vi "testDisplay.vi"() -> ()   [LabVIEW 2017]
panel:
  out "projBounds":T1
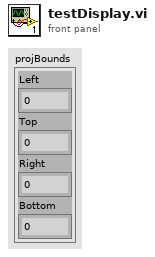
[diagram p1: front panel]
types:
  T1 = cluster{"Left":i32, "Top":i32, "Right":i32, "Bottom":i32}
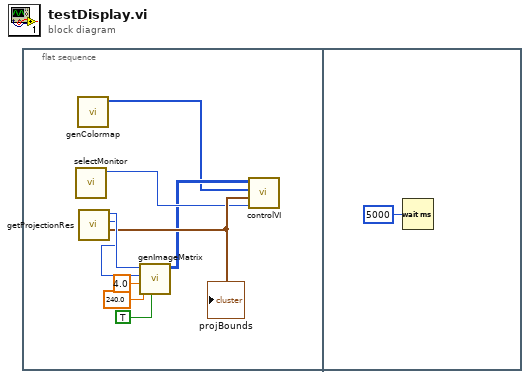
[diagram p0: block diagram]
diagram:
  n1 = flat-sequence {
    frame #0 {
      n2 = call "selectMonitor.vi"() -> ("monitor to use"=w4:i32)  [unwired: 11 in]
      n3 = call "genColormap.vi"() -> ("Colormap"=w2:u32[])  [unwired: 11 in]
      n4 = call "getProjectionRes.vi"() -> ("projBounds"=w5:T1, "YRes"=w8:i32, "XRes"=w9:i32)  [unwired: 9 in]
      "projBounds" <- w5
      n5 = call "genImageMatrix.vi"("Orientation"=TRUE, "Phase"=240.0, "Cycles"=4.0, "Y resolution"=w8, "X Resolution"=w9) -> ("Scan Image"=w3:u8[][])  [unwired: 5 in, 1 out]
      n6 = call "controlVI.vi"("monitorToUse"=w4, "Front Panel Window:Window Bounds"=w5, "colors"=w2, "8-bit pixmap"=w3) -> ()  [unwired: 7 in, 1 out]
    }
    frame #1 {
      n7 = Wait (ms)(milliseconds to wait=u32 5000) -> ()  [unwired: 1 out]
    }
  }
